vi "Interface.vi"(8 "error in (no error)":errorcluster) -> (0 "error out":errorcluster)   [LabVIEW 2016]
uses:
  <vilib>/Platform/TimedLoop/XDataNode/timing_clust.ctl
  <vilib>/Platform/TimedLoop/XDataNode/nitl_modes.ctl
  <vilib>/Platform/TimedLoop/XDataNode/wakeup.ctl
  <vilib>/Platform/TimedLoop/XDataNode/XDataNode.xnode
  <vilib>/Platform/TimedLoop/XDataNode/XDNodeRunTimeDep.lvlib
  <vilib>/GoldZinc Software/auzn custom VIs/CustomVI.lvlib
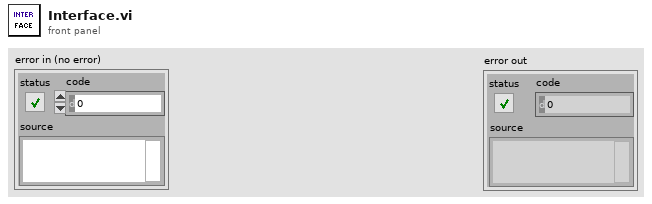
[diagram p1: front panel]
types:
  T1 = typedef "XDNodeRunTimeDep.lvlib/timing_clust.ctl" = cluster{"Expected End [f-1]":u64, "Actual End [f-1]":u64, "Finished Late? [f-1]":bool, "Expected End [i-1]":u64, "Actual End [i-1]":u64, "Finished Late? [i-1]":bool, "Expected Start [i]":u64, "Actual Start [i]":u64, "Expected Start [f]":u64, "Actual Start [f]":u64, "Source Name":string, "Structure Name":string, "Period":i64, "Deadline":i64, "Offset":i64, "Start":i64, "Priority":i32, "Timeout":i32, "Mode":T2, "Wakeup Reason":T3, "Error":errorcluster, "Source Type":string, "Secondary Source Type":string, "Global End Time":u64, "Global Start Time":u64, "Frame Duration":u64, "Iteration Duration":u64, "Assigned CPU":i32, "I/O Scan Engine Mode":u32}
  T2 = typedef "XDNodeRunTimeDep.lvlib/nitl_modes.ctl" = enum32{"No Change", "Process missed periods, maintain original phase", "Discard missed periods, maintain original phase", "Process missed periods, ignore original phase", "Discard missed periods, ignore original phase"}
  T3 = typedef "XDNodeRunTimeDep.lvlib/wakeup.ctl" = enum32{"Normal", "Aborted", "Asynchronous wakeup", "Timing source error", "Timed loop error", "Timeout"}
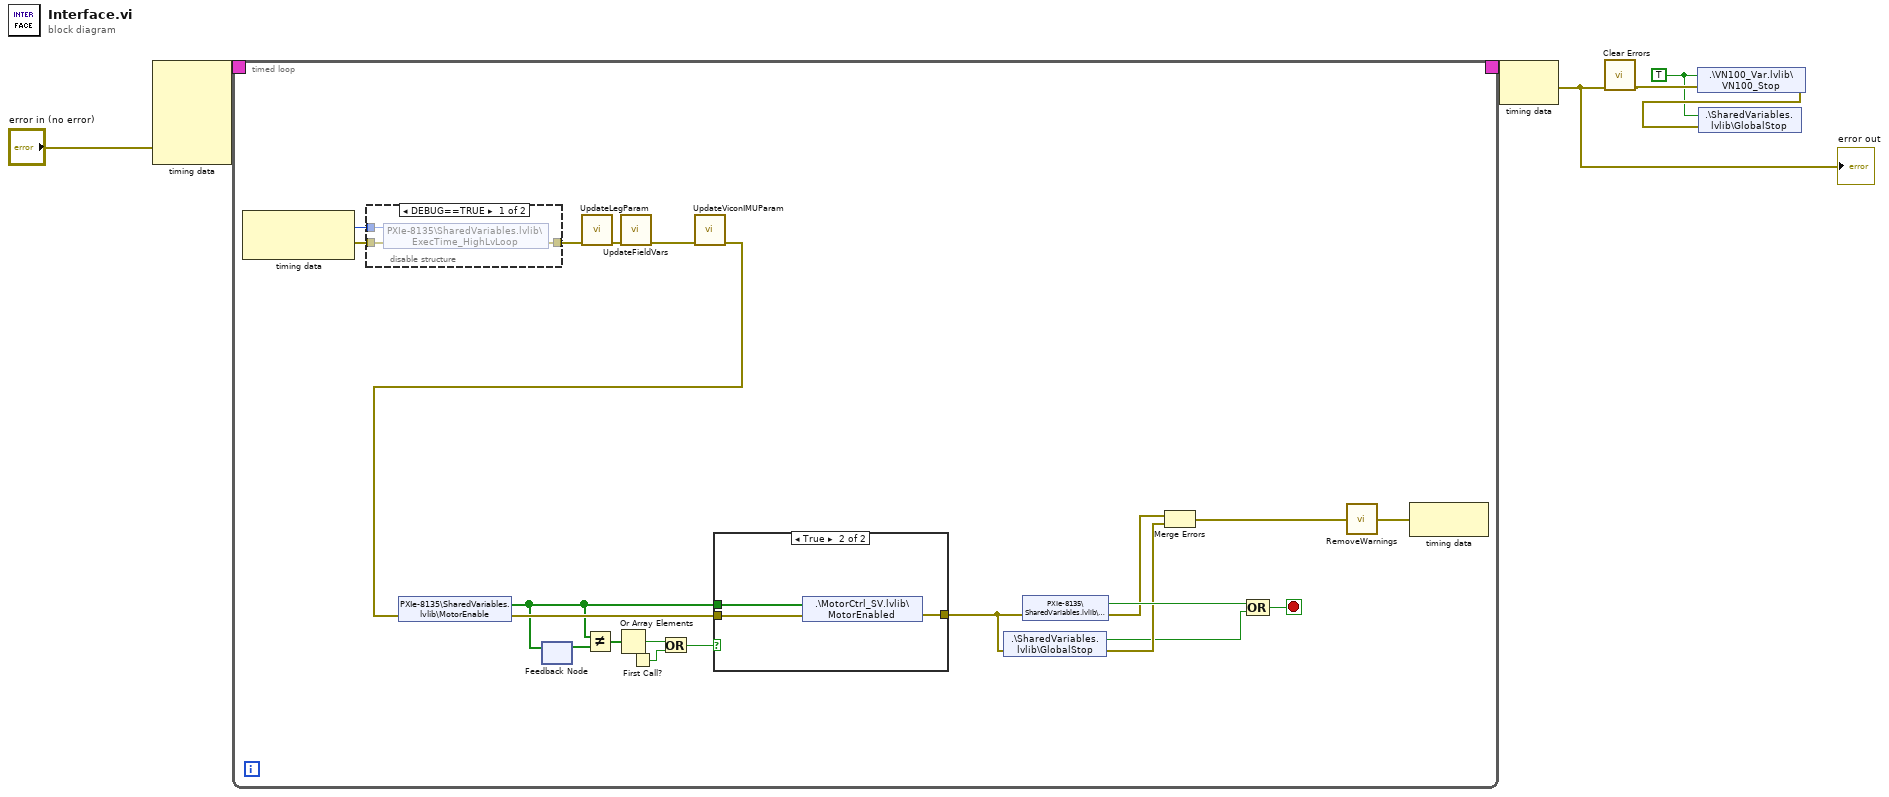
[diagram p0: block diagram]
diagram:
  w1 = TRUE ("VN100_Stop")
  n1 = node-c288("error in (no error)") -> (w7:T1)  [unwired: 4 in]
  n2 = timed-loop {
    timing: w7 -> [_]
    timing-out: [_] -> w6
    stop <- w17 stop-if-true
    n3 = node-c288() -> (w19:i64, w12:errorcluster)  [unwired: 1 in]
    n4 = disable-structure shown="DEBUG==TRUE" {
      disable-tunnel: w19 -> [w31 _]
      disable-tunnel: w12 -> [w30 w32]
      disable-tunnel: [w29 w32] -> w11
      frame condition #0 {
        n5 = shared-variable "PXIe-8135\\SharedVariables.lvlib\\ExecTime_HighLvLoop"(w31, error in=w30) -> (error out=w29:errorcluster)
      }
      frame condition #1 (active) {
      }
    }
    n6 = feedback #1() -> (w25:bool[])  [unwired: 1 in]
    n7 = call "UpdateLegParam.vi"("error in (no error)"=w11) -> ("error out"=w28:errorcluster)  [unwired: 10 in]
    n8 = call "UpdateFieldVars.vi"("error in (no error)"=w28) -> ("error out"=w8:errorcluster)  [unwired: 10 in]
    n9 = First Call?() -> (First Call?: T/F=w20:bool)
    n10 = call "UpdateViconIMUParam.vi"("error in (no error)"=w8) -> ("error out"=w27:errorcluster)  [unwired: 10 in]
    n11 = shared-variable "PXIe-8135\\SharedVariables.lvlib\\MotorEnable"(error in=w27) -> (w23:bool[], error out=w26:errorcluster)
    n12 = feedback-in #1(w23) -> ()
    n13 = Not Equal?(x=w23, y=w25) -> (x != y?=w24:bool[])
    n14 = Or Array Elements(Boolean array=w24) -> (logical OR=w22:bool)
    n15 = Or(x=w22, y=w20) -> (x .or. y?=w21:bool)
    n16 = case shown="True" w21 {
      tunnel: w26 -> [w33 w36]
      tunnel: w23 -> [_ w34]
      tunnel: [w33 w35] -> w16
      frame False {
      }
      frame True {
        n17 = shared-variable ".\\MotorCtrl_SV.lvlib\\MotorEnabled"(w34, error in=w36) -> (error out=w35:errorcluster)
      }
    }
    n18 = shared-variable ".\\SharedVariables.lvlib\\GlobalStop"(error in=w16) -> (w13:bool, error out=w14:errorcluster)
    n19 = shared-variable "PXIe-8135\\SharedVariables.lvlib\\Stop RT"(error in=w16) -> (w18:bool, error out=w15:errorcluster)
    n20 = Merge Errors(w15, w14) -> (w9:errorcluster)
    n21 = Compound Arithmetic op=OR(w18, w13) -> (w17:bool)
    n22 = call <vilib>:"RemoveWarnings.vi"("error in (no error)"=w9) -> ("error out"=w10:errorcluster)
    n23 = node-c288(w10) -> ()  [unwired: 1 out]
  }
  n24 = node-c288(w6) -> (w2:errorcluster)
  "error out" <- w2
  n25 = call <vilib>:"Clear Errors.vi"("error in (no error)"=w2) -> ("error out"=w3:errorcluster)  [unwired: 5 in, 1 out]
  n26 = shared-variable ".\\VN100_Var.lvlib\\VN100_Stop"(w1, error in=w3) -> (error out=w4:errorcluster)
  n27 = shared-variable ".\\SharedVariables.lvlib\\GlobalStop"(w1, error in=w4) -> ()  [unwired: 1 out]
